vi "TEMP STAB.vi"(0 "Queue in":refnum<queue>, 1 "element in":T1 {"Output's Control Loop (1:1)" items=["1"=1, "2"=2]; "Data Source (0:Kelvin)" items=["Kelvin", "Celsius", "Sensor Units"]; "Input (0:A)" items=["A", "B", "C", "D", "D2", "D3", "D4", "D5"]; "Configure Control Parameters (0: Configure)" items=["Configure", "Don't Configure"]; "Serial Configuration"."Flow Control" items=["None", "XON/XOFF", "RTS/CTS", "XON/XOFF & RTS/CTS", "DTR/DSR", "XON/XOFF & DTR/DSR"]; "Serial Configuration"."Stop Bits" items=["1.0"=10, "1.5"=15, "2.0"=20]; "Serial Configuration"."Data Bits" items=["7"=7, "8"=8]; "Serial Configuration"."Parity" items=["None", "Odd", "Even", "Mark", "Space"]; "Serial Configuration"."Baud Rate" items=["300"=300, "600"=600, "1200"=1200, "2400"=2400, "4800"=4800, "9600"=9600, "19200"=19200, "38400"=38400, "57600"=57600]; "Target Temp (K)" format="%.5f"; "Input (0:None)" items=["None", "A", "B", "C", "D", "D2", "D3", "D4", "D5"]; "Mode (0:Off)" items=["Off", "Closed Loop PID", "Zone", "Open Loop"]; "Heater Out Display (1:Current)" items=["Current"=1, "Power"=2]; "Max Current (0:User Specified)" items=["User Specified", "0.707 A", "1.0 A", "1.141 A", "2.0 A"]; "Heater Resistance (1:25 Ohms)" items=["25 Ohms"=1, "50 Ohms"=2]; "Max User Current (2.000)" format="%.3f"; "Gain (P) (50.0)" format="%.1f"; "Reset (I) (20.0)" format="%.1f"; "Rate (D) (0.0 %)" format="%.1f"; "Manual Output (0.00 %)" format="%.2f"; "Range (0:Off)" items=["Off", "Range 1 (On)", "Range 2", "Range 3", "Range 4", "Range 5"]}, 5 "Array in":dbl[](array[numeric]), 7 "ScanQ In":refnum<queue>, 9 "Setpoint":dbl, 11 "error in (no error)":errorcluster) -> (4 "Queue out":refnum<queue>, 6 "Array out":dbl[](array[numeric]), 8 "ScanQ":refnum<queue>, 10 "element out":T1 {"Output's Control Loop (1:1)" items=["1"=1, "2"=2]; "Data Source (0:Kelvin)" items=["Kelvin", "Celsius", "Sensor Units"]; "Input (0:A)" items=["A", "B", "C", "D", "D2", "D3", "D4", "D5"]; "Configure Control Parameters (0: Configure)" items=["Configure", "Don't Configure"]; "Serial Configuration"."Flow Control" items=["None", "XON/XOFF", "RTS/CTS", "XON/XOFF & RTS/CTS", "DTR/DSR", "XON/XOFF & DTR/DSR"]; "Serial Configuration"."Stop Bits" items=["1.0"=10, "1.5"=15, "2.0"=20]; "Serial Configuration"."Data Bits" items=["7"=7, "8"=8]; "Serial Configuration"."Parity" items=["None", "Odd", "Even", "Mark", "Space"]; "Serial Configuration"."Baud Rate" items=["300"=300, "600"=600, "1200"=1200, "2400"=2400, "4800"=4800, "9600"=9600, "19200"=19200, "38400"=38400, "57600"=57600]; "Target Temp (K)" format="%.5f"; "Input (0:None)" items=["None", "A", "B", "C", "D", "D2", "D3", "D4", "D5"]; "Mode (0:Off)" items=["Off", "Closed Loop PID", "Zone", "Open Loop"]; "Heater Out Display (1:Current)" items=["Current"=1, "Power"=2]; "Max Current (0:User Specified)" items=["User Specified", "0.707 A", "1.0 A", "1.141 A", "2.0 A"]; "Heater Resistance (1:25 Ohms)" items=["25 Ohms"=1, "50 Ohms"=2]; "Max User Current (2.000)" format="%.3f"; "Gain (P) (50.0)" format="%.1f"; "Reset (I) (20.0)" format="%.1f"; "Rate (D) (0.0 %)" format="%.1f"; "Manual Output (0.00 %)" format="%.2f"; "Range (0:Off)" items=["Off", "Range 1 (On)", "Range 2", "Range 3", "Range 4", "Range 5"]}, 15 "error out":errorcluster)   [LabVIEW 2025]
uses:
  Downloads/OneDrive_2025-09-03/Instrument Controls/Temp Cntrl.ctl
  STM-Auto-Project/QMH CTLS/Scan_Params (QMH).ctl
  <vilib>/Analysis/baseanly.llb/Mean (DBL).vi
  <vilib>/Analysis/NI_AALBase.lvlib
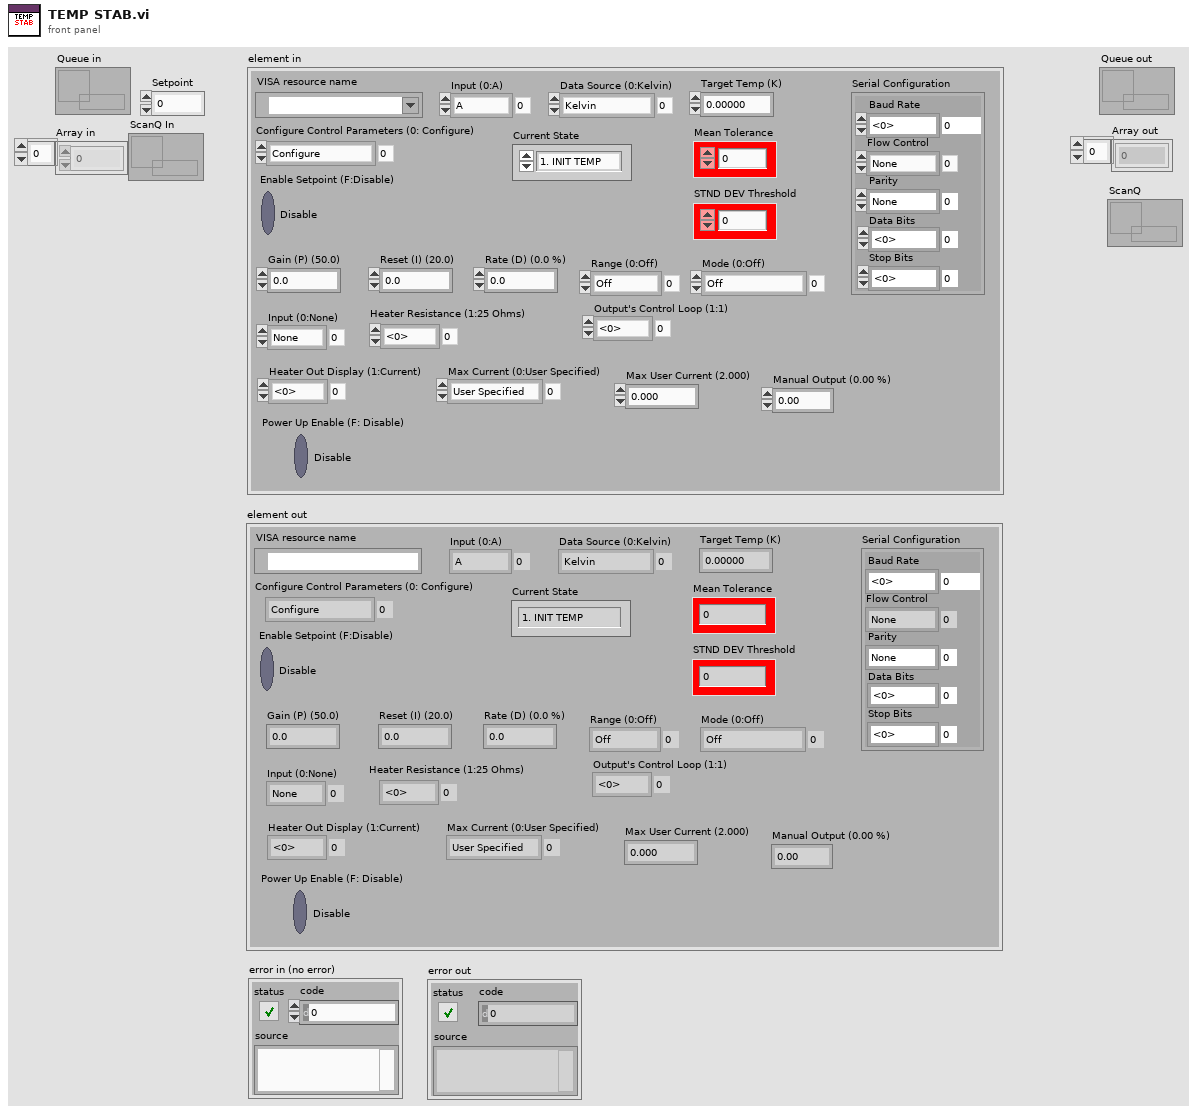
[diagram p1: front panel]
types:
  T1 = typedef "Temp Cntrl.ctl" = cluster{"Range (0:Off)":u16, "Manual Output (0.00 %)":dbl, "Rate (D) (0.0 %)":dbl, "Reset (I) (20.0)":dbl, "Gain (P) (50.0)":dbl, "Power Up Enable (F: Disable)":bool, "Max User Current (2.000)":dbl, "Heater Resistance (1:25 Ohms)":u16, "Max Current (0:User Specified)":u16, "Heater Out Display (1:Current)":u16, "Mode (0:Off)":u16, "Input (0:None)":u16, "Target Temp (K)":dbl, "Serial Configuration":cluster{"Baud Rate":u32, "Parity":u16, "Data Bits":u16, "Stop Bits":u16, "Flow Control":u16}, "VISA resource name":refnum<visa-resource-name>, "Configure Control Parameters (0: Configure)":u16, "Enable Setpoint (F:Disable)":bool, "Input (0:A)":u16, "Data Source (0:Kelvin)":u16, "Output's Control Loop (1:1)":u16, "STND DEV Threshold ":dbl, "Mean Tolerance ":dbl, "Current State":enum16{"1. INIT TEMP", "2. TC ON", "3. POLL_TEMPS", "4. TEMP_STAB", "5. TC IDLE", "6. APPLY NEXT TEMP", "7. TC OFF (Reset)"}}
  T2 = enum16{"1. INIT TEMP", "2. TC ON", "3. POLL_TEMPS", "4. TEMP_STAB", "5. TC IDLE", "6. APPLY NEXT TEMP", "7. TC OFF (Reset)"}
  T3 = enum16{"1. BIAS", "2. INIT_SCAN", "3. SCAN_IDLE", "4. INTER_SCAN", "5. NEW_COORDS_&_FRAME", "6. FINAL_SCAN", "7. POLL BIAS ", "8. Z-CONT.", "9. STOP"}
  T4 = typedef "Scan_Params (QMH).ctl" = cluster{"Setpoint (I)":dbl[], "Bias (V)":dbl[], "Number of scans":u8, "Port number (3364)":u32, "Avoid zero threshold (V)":dbl, "Current State":enum16{"1. BIAS", "2. INIT_SCAN", "3. SCAN_IDLE", "4. INTER_SCAN", "5. NEW_COORDS_&_FRAME", "6. FINAL_SCAN", "7. POLL BIAS ", "8. Z-CONT.", "9. STOP"}}
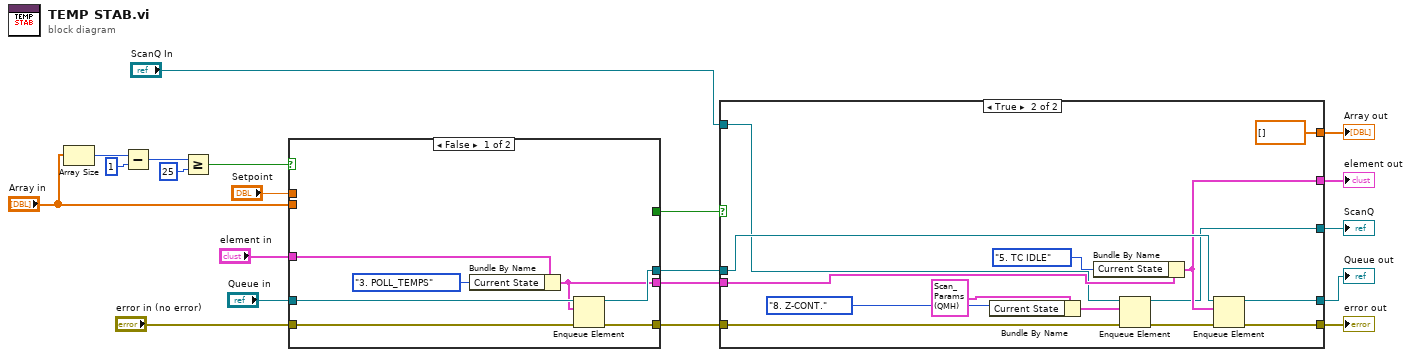
[diagram p0: block diagram]
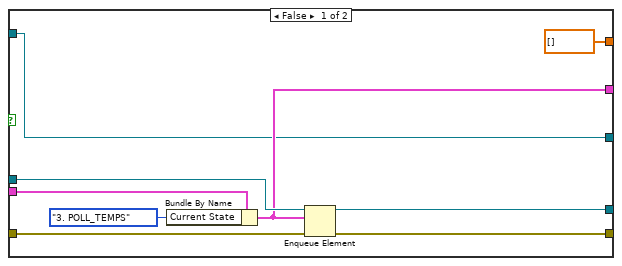
[diagram p2: hidden frame]
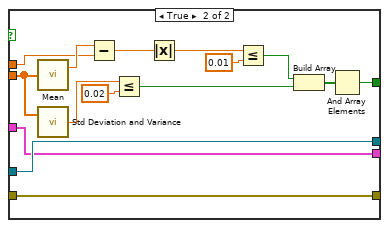
[diagram p3: hidden frame]
diagram:
  n1 = Array Size(array="Array in") -> (size(s)=w3:i32)
  n2 = Subtract(x=w3, y=1) -> (x-y=w5:i32)
  n3 = Greater Or Equal?(x=w5, y=25) -> (x >= y?=w7:bool)
  n4 = case shown="False" w7 {
    tunnel: "Setpoint" -> [_ w38]
    tunnel: "Array in" -> [_ w33]
    tunnel: [_ w31] -> w12
    tunnel: "Queue in" -> [w27 w30]
    tunnel: "element in" -> [w26 w29]
    tunnel: "error in (no error)" -> [w25 w28]
    tunnel: [w24 w30] -> w13
    tunnel: [w23 w28] -> w14
    tunnel: [w22 w29] -> w15
    frame False {
      n5 = Bundle By Name(cluster=w26, "Current State"=T2."3. POLL_TEMPS") -> (w22:T1)
      n6 = Enqueue Element(queue=w27, element=w22, error in (no error)=w25) -> (queue out=w24:refnum<queue>, error out=w23:errorcluster)  [unwired: 1 in, 1 out]
    }
    frame True {
      n7 = call-poly <vilib>:"Mean.vi"("X"=w33) -> ("mean"=w40:dbl)  [unwired: 1 out]
      n8 = call <vilib>:"Std Deviation and Variance.vi"("X"=w33) -> ("standard deviation"=w42:dbl)  [unwired: 1 in, 2 out]
      n9 = Subtract(x=w40, y=w38) -> (x-y=w39:dbl)
      n10 = Less Or Equal?(x=w42, y=0.02) -> (x <= y?=w34:bool)
      n11 = Absolute Value(x=w39) -> (abs(x)=w37:dbl)
      n12 = Less Or Equal?(x=w37, y=0.01) -> (x <= y?=w35:bool)
      n13 = Build Array(w35, w34) -> (w32:bool[])
      n14 = And Array Elements(Boolean array=w32) -> (logical AND=w31:bool)
    }
  }
  n15 = case shown="True" w12 {
    tunnel: w13 -> [w50 w65]
    tunnel: w14 -> [w46 w55]
    tunnel: w15 -> [w49 w64]
    tunnel: [w48 w63] -> w16
    tunnel: [w47 w62] -> w17
    tunnel: [dbl[] [] dbl[] []] -> w18
    tunnel: [w45 w60] -> w20
    tunnel: "ScanQ In" -> [w44 w59]
    tunnel: [w44 w56] -> w2
    frame False {
      n16 = Bundle By Name(cluster=w49, "Current State"=T2."3. POLL_TEMPS") -> (w45:T1)
      n17 = Enqueue Element(queue=w50, element=w45, error in (no error)=w46) -> (queue out=w48:refnum<queue>, error out=w47:errorcluster)  [unwired: 1 in, 1 out]
    }
    frame True {
      n18 = Bundle By Name(cluster=T4 {"Setpoint (I)"=[], "Bias (V)"=[], "Number of scans"=1, "Port number (3364)"=3364, "Avoid zero threshold (V)"=0.004999999888241291, "Current State"=enum."1. BIAS"} ("element"), "Current State"=T3."8. Z-CONT.") -> (w57:T4)
      n19 = Bundle By Name(cluster=w64, "Current State"=T2."5. TC IDLE") -> (w60:T1)
      n20 = Enqueue Element(queue=w59, element=w57, error in (no error)=w55) -> (queue out=w56:refnum<queue>, error out=w54:errorcluster)  [unwired: 1 in, 1 out]
      n21 = Enqueue Element(queue=w65, element=w60, error in (no error)=w54) -> (queue out=w63:refnum<queue>, error out=w62:errorcluster)  [unwired: 1 in, 1 out]
    }
  }
  "element out" <- w20
  "Array out" <- w18
  "error out" <- w17
  "Queue out" <- w16
  "ScanQ" <- w2
